vi "SwissSPAD Live_Q Name Conversion.vi"(11 "SwissSPAD Live Gate Data Decode Q Name":string) -> (3 "FPGA Q Name":string)   [LabVIEW 2021]
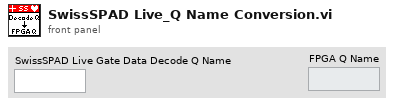
[diagram p1: front panel]
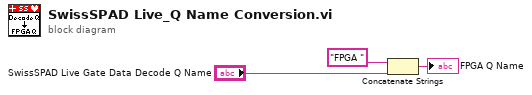
[diagram p0: block diagram]
diagram:
  n1 = Concatenate Strings("FPGA " ("string"), "SwissSPAD Live Gate Data Decode Q Name") -> (→"FPGA Q Name":string)
